vi "GetStaleStreamsFromDisk.vi"(8 "error in (no error)":errorcluster) -> (0 "error out":errorcluster, 3 "streams":variant)   [LabVIEW 2017, in "FileManager.lvlib"]
uses:
  <vilib>/addons/InsightCM/Devices/Shared/Common/FileManager/FileManager.lvlib
  <vilib>/addons/InsightCM/Devices/Shared/Common/FileManager/controls/StreamState.ctl
  <vilib>/addons/InsightCM/Utilities/GlobalConfiguration/GlobalConfiguration.lvlib
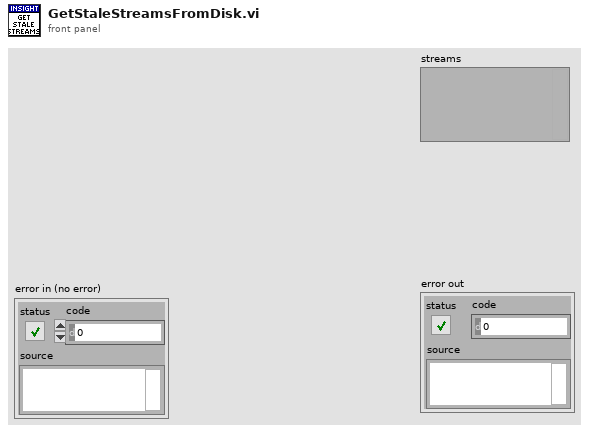
[diagram p1: front panel]
types:
  T1 = typedef "FileManager.lvlib/StreamState.ctl" = cluster{"DataGroup":string, "Stream Id":string, "LastBlock":bool, "TotalBlocks":i32, "BlocksSent":i32, "Device":string}
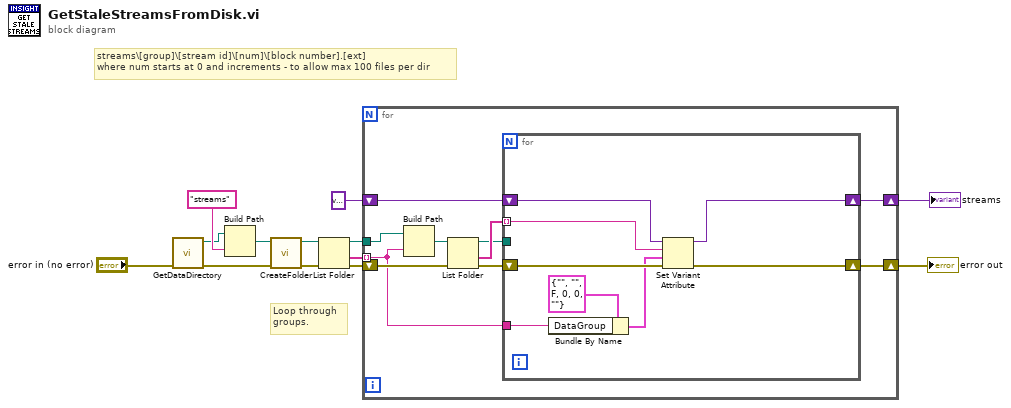
[diagram p0: block diagram]
diagram:
  # "Loop through\ngroups."
  # "streams\\[group]\\[stream id]\\[num]\\[block number].[ext]\nwhere num starts at 0 and increments - to allow max 100 files per dir"
  n1 = call <vilib>:"GetDataDirectory.vi"("error in (no error)"="error in (no error)") -> ("error out"=w1:errorcluster, "data directory"=w3:path)  [unwired: 9 in]
  n2 = Build Path(base path=w3, name or relative path="streams") -> (appended path=w9:path)
  n3 = call <vilib>:"CreateFolder.vi"("error in (no error)"=w1, "folder"=w9) -> ("error out"=w8:errorcluster, "folder out"=w6:path)  [unwired: 8 in]
  n4 = List Folder(path=w6, error in=w8) -> (path out=w5:path, folder names=w4:string[], error out=w7:errorcluster)  [unwired: 1 in, 2 out]
  n5 = for {
    shift-right: [w18] -> w11
    shift-left: variant ("variant") -> [w21]
    shift-right: [w23] -> w13
    shift-left: w7 -> [w17]
    tunnel: w5 -> [w16]
    tunnel: w4 -> [w14] mode=indexing
    n6 = Build Path(base path=w16, name or relative path=w14) -> (appended path=w15:path)
    n7 = List Folder(path=w15, error in=w17) -> (path out=w19:path, folder names=w20:string[], error out=w22:errorcluster)  [unwired: 1 in, 2 out]
    n8 = for {
      shift-right: [w31] -> w23
      shift-left: w22 -> [w27]
      shift-right: [w29] -> w18
      shift-left: w21 -> [w30]
      tunnel: w20 -> [w26] mode=indexing
      tunnel: w19 -> [_]
      tunnel: w14 -> [w28]
      n9 = Bundle By Name(cluster=T1 {"DataGroup"="", "Stream Id"="", "LastBlock"=FALSE, "TotalBlocks"=0, "BlocksSent"=0, "Device"=""} ("Stream"), "DataGroup"=w28) -> (w24:T1)
      n10 = Set Variant Attribute(Variant=w30, name=w26, value=w24, error in=w27) -> (Variant out=w29:variant, error out=w31:errorcluster)  [unwired: 1 out]
    }
  }
  "error out" <- w13
  "streams" <- w11
